vi "NI VeriStand - Get Channel FIFO Buffer Index.vi"(8 "error in":errorcluster, 10 "Channel Ref":T2 format="%.0x", 11 "Device Ref in":T2 format="%.0x") -> (0 "error out":errorcluster, 2 "Channel FIFO Buffer Index":i32, 3 "Device Ref out":T2 format="%.0x", 4 "Found":bool, 5 "FIFO Buffer":T1)   [LabVIEW 2020, in "Custom Device Utility Library.lvlib"]
doc: "Gets the FIFO buffer index for the custom device channel specified by <B>Channel Ref</B> and determines which <B>FIFO Buffer</B> (input or output) contains the channel. Use this VI to determine which index to read or write a channel value to in the FIFO arrays for an asynchronous custom device.\n\nUse this VI with channels of asynchronous custom devices only."
uses:
  <vilib>/NI VeriStand/Custom Device Tools/Custom Device Utility Library/Custom Device Utility Library.lvlib
  <vilib>/NI VeriStand/Custom Device API/Custom Device Item Ref.ctl
  <vilib>/NI VeriStand/Custom Device API/Custom Device Channel Type.ctl
  <vilib>/NI VeriStand/Custom Device API/Custom Device API.lvlib
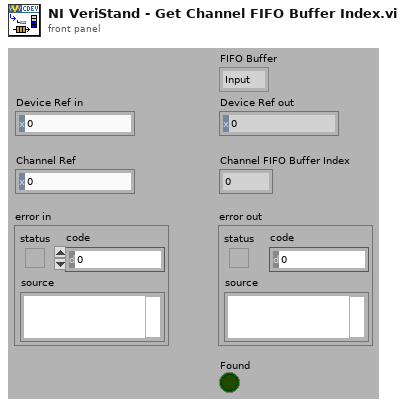
[diagram p1: front panel]
types:
  T1 = typedef "Custom Device API.lvlib/Custom Device Channel Type.ctl" = enum16{"Input", "Output"}
  T2 = typedef "Custom Device API.lvlib/Custom Device Item Ref.ctl" = u64
  T3 = typedef "Custom Device API.lvlib/Custom Device Channel.ctl" = cluster{"Type":T1, "Units":string, "Default Value":dbl, "Faultable":bool, "Scalable":bool}
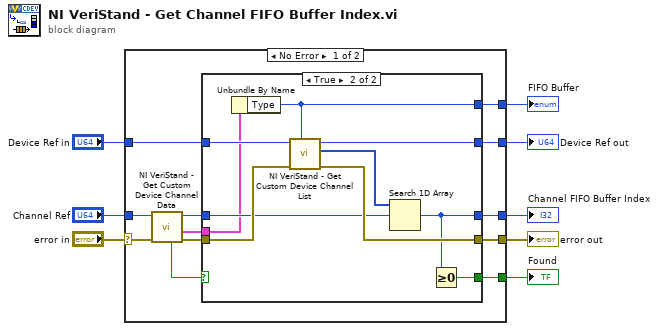
[diagram p0: block diagram]
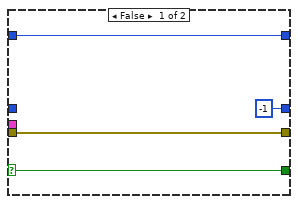
[diagram p2: hidden frame]
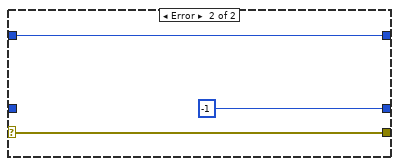
[diagram p3: hidden frame]
diagram:
  n1 = case shown="No Error" "error in" {
    selector: "error in" -> [w12 w35]
    tunnel: [w19 w35] -> w8
    tunnel: [w17 w36] -> w7
    tunnel: [w11 -1 ("index of element")] -> w6
    tunnel: "Channel Ref" -> [w15 _]
    tunnel: [w14 _] -> w4
    tunnel: "Device Ref in" -> [w20 w36]
    tunnel: [w10 _] -> w1
    frame No Error {
      n2 = call <vilib>:"NI VeriStand - Get Custom Device Channel Data.vi"("error in (no error)"=w12, "Channel Ref in"=w15) -> ("error out"=w18:errorcluster, "Channel"=w13:T3, "Channel Ref out"=w16:T2, "Found"=w9:bool)  [unwired: 6 out]
      n3 = case shown="True" w9 {
        selector: w9 -> [w21 _]
        tunnel: w20 -> [w24 w34]
        tunnel: [w22 w33] -> w19
        tunnel: w18 -> [w22 w32]
        tunnel: [w24 w31] -> w17
        tunnel: w16 -> [_ w30]
        tunnel: [_ w28] -> w14
        tunnel: w13 -> [_ w27]
        tunnel: [-1 ("index of element") w26] -> w11
        tunnel: [w21 w25] -> w10
        frame False {
        }
        frame True {
          n4 = Unbundle By Name(w27) -> ("Type"=w28:T1)
          n5 = call <vilib>:"NI VeriStand - Get Custom Device Channel List.vi"("Channel Type"=w28, "error in (no error)"=w32, "Device Ref in"=w34) -> ("error out"=w33:errorcluster, "Specified Channel Ref List"=w29:T2[], "Device Ref out"=w31:T2)  [unwired: 6 out]
          n6 = Search 1D Array(1D array=w29, element=w30) -> (index of element=w26:i32)  [unwired: 1 out]
          n7 = Greater Or Equal To 0?(x=w26) -> (x >= 0?=w25:bool)
        }
      }
    }
    frame Error {
    }
  }
  "Device Ref out" <- w7
  "Channel FIFO Buffer Index" <- w6
  "error out" <- w8
  "FIFO Buffer" <- w4
  "Found" <- w1
